vi "Duration Calculation.vi"(8 "error in (no error)":errorcluster, 10 "Breakdown out time":string[](array[string]), 11 "Breakdown in time":string[](array[string])) -> (0 "error out":errorcluster, 2 "Array 2":string[](array[string]), 3 "DURATION":dbl, 5 "Array":dbl[](array[numeric]))   [LabVIEW 2017]
panel:
  # "2020-09-07 22:56:14"
  # "2020-09-08 0:06:51"
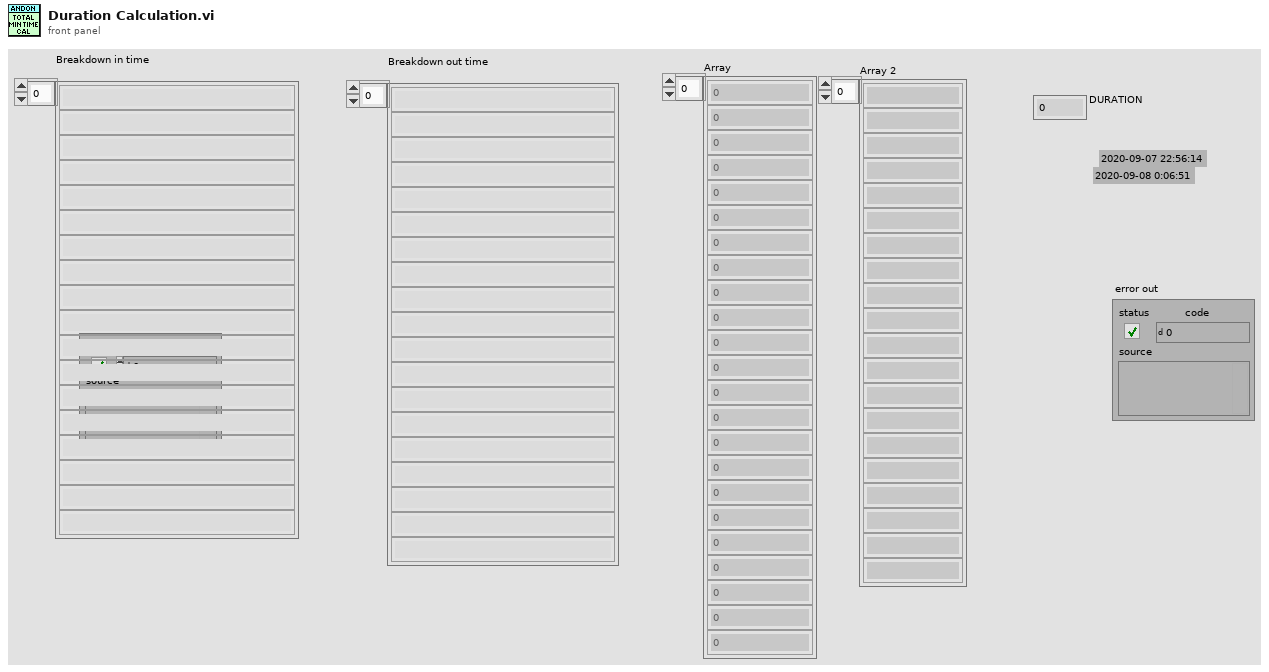
[diagram p1: front panel]
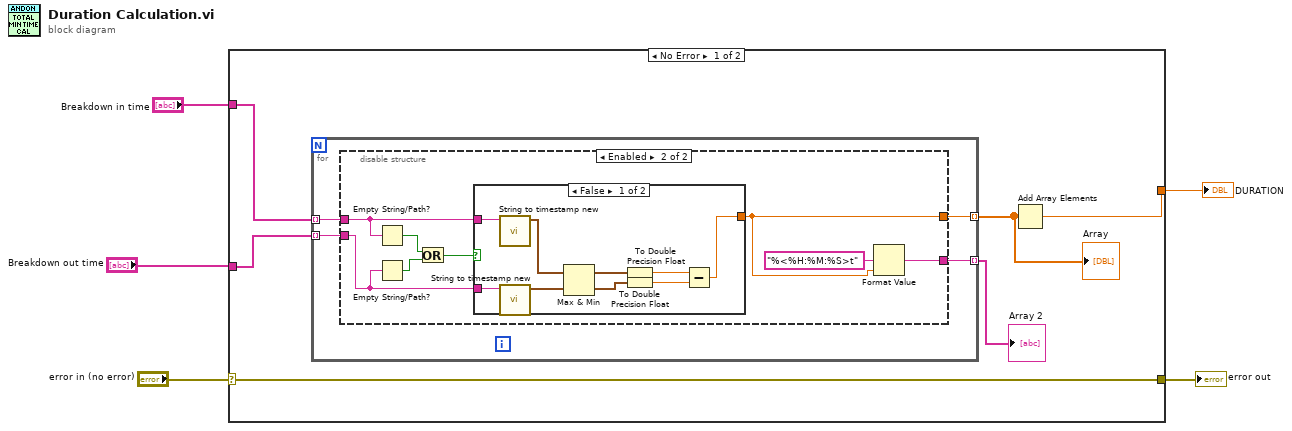
[diagram p0: block diagram]
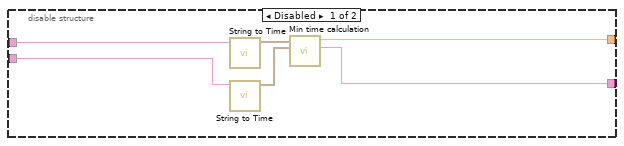
[diagram p2: hidden frame]
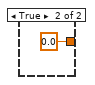
[diagram p3: hidden frame]
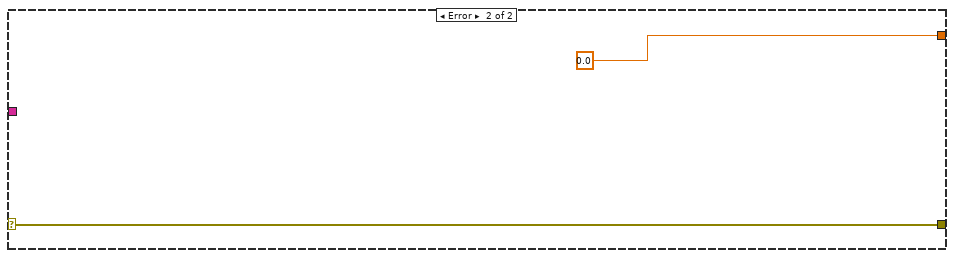
[diagram p4: hidden frame]
diagram:
  n1 = case shown="No Error" "error in (no error)" {
    selector: "error in (no error)" -> [w10 w41]
    tunnel: [w10 w41] -> w3
    tunnel: [w9 0.0] -> w4
    tunnel: "Breakdown in time" -> [w8 _]
    tunnel: "Breakdown out time" -> [w7 _]
    frame No Error {
      n2 = for {
        tunnel: w8 -> [w15] mode=indexing
        tunnel: w7 -> [w14] mode=indexing
        tunnel: [w13] -> w11 mode=indexing
        tunnel: [w12] -> w6 mode=indexing
        n3 = disable-structure shown="Enabled" {
          disable-tunnel: w15 -> [w21 w26]
          disable-tunnel: w14 -> [w20 w25]
          disable-tunnel: [w17 w27] -> w13
          disable-tunnel: [w16 w28] -> w12
          frame Disabled {
            n4 = call "String to Time.vi"("String"=w21) -> ("Time Stamp"=w19:timestamp)  [unwired: 9 in, 1 out]
            n5 = call "String to Time.vi"("String"=w20) -> ("Time Stamp"=w18:timestamp)  [unwired: 9 in, 1 out]
            n6 = call "Min time calculation.vi"("Breakdown out Time Stamp"=w18, "Breakdown inTime Stamp"=w19) -> ("Time"=w16:string, "min"=w17:dbl)  [unwired: 7 in, 1 out]
          }
          frame Enabled {
            n7 = Empty String/Path?(string/path=w26) -> (empty?=w23:bool)
            n8 = Empty String/Path?(string/path=w25) -> (empty?=w24:bool)
            n9 = Or(x=w23, y=w24) -> (x .or. y?=w22:bool)
            n10 = case shown="False" w22 {
              tunnel: [w32 0.0] -> w27
              tunnel: w26 -> [w31 _]
              tunnel: w25 -> [w30 _]
              frame False {
                n11 = call "String to timestamp new.vi"("String Timestamp"=w31) -> ("Timestamp"=w34:timestamp)  [unwired: 10 in]
                n12 = call "String to timestamp new.vi"("String Timestamp"=w30) -> ("Timestamp"=w33:timestamp)  [unwired: 10 in]
                n13 = Max & Min(x=w34, y=w33) -> (max(x,y)=w38:timestamp, min(x,y)=w37:timestamp)
                n14 = To Double Precision Float(number=w38) -> (double precision float=w36:dbl)
                n15 = To Double Precision Float(number=w37) -> (double precision float=w35:dbl)
                n16 = Subtract(x=w36, y=w35) -> (x-y=w32:dbl)
              }
              frame True {
              }
            }
            n17 = Format Value(format string="%<%H:%M:%S>t", value (0)=w27) -> (output string=w28:string)  [unwired: 1 in]
          }
        }
      }
      "Array" <- w11
      "Array 2" <- w6
      n18 = Add Array Elements(numeric array=w11) -> (sum=w9:dbl)
    }
    frame Error {
    }
  }
  "error out" <- w3
  "DURATION" <- w4
